vi "4Linea.vi"() -> ()   [LabVIEW 2020]
panel:
  out "Nadie Gana":bool
  in  "OK Button":bool
  out "4Linea":string[][](array[string])
  out "Turno de":string
  in  "Turno de":bool
  out "X Gana T":bool
  in  "Arreglo4Linea":bool[][](array[boolean])=[[FALSE, FALSE, FALSE], [FALSE, FALSE, FALSE], [FALSE, FALSE, FALSE]]
  out "O Gana T":bool
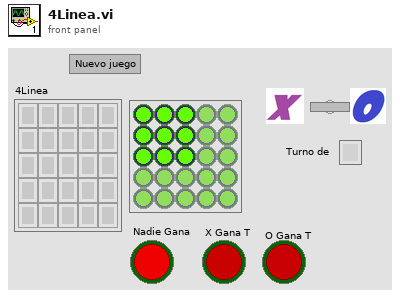
[diagram p1: front panel]
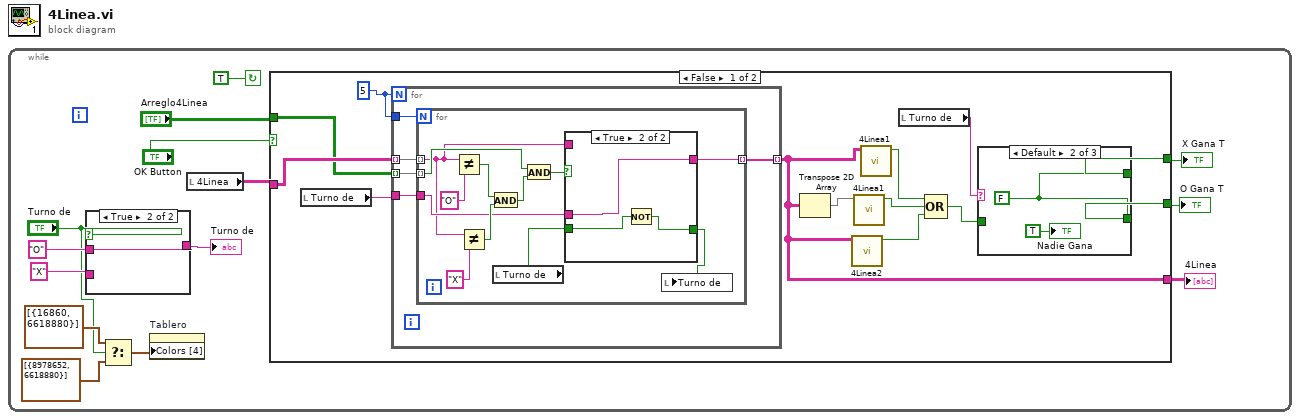
[diagram p0: block diagram]
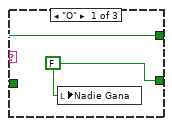
[diagram p3: hidden frame]
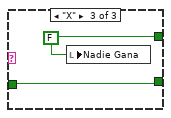
[diagram p4: hidden frame]
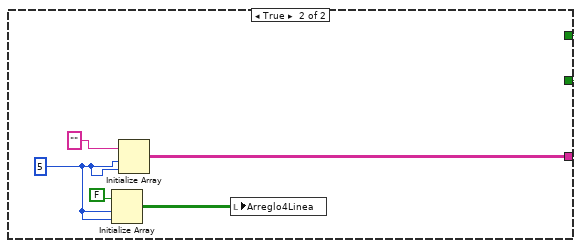
[diagram p6: hidden frame]
diagram:
  n1 = while {
    stop <- TRUE continue-if-true
    n2 = case shown="True" "Turno de" {
      tunnel: "O" -> [_ w16]
      tunnel: "X" -> [w15 _]
      tunnel: [w15 w16] -> w11
      frame False {
      }
      frame True {
      }
    }
    "Turno de" <- w11
    n3 = Select(t=cluster{u32, u32}[] [{16860, 6618880}] ("Colors [4]"), s="Turno de", f=cluster{u32, u32}[] [{8978652, 6618880}] ("Colors [4]")) -> (s? t:f=w1:cluster{u32, u32}[])
    n4 = property on="Tablero" class="Bool (strict)"("Colors [4]"=w1) -> ()  [unwired: 2 in, 2 out]
    n5 = local read "4Linea"() -> (w14:string[][])
    n6 = case shown="False" "OK Button" {
      tunnel: [w17 w65] -> w8
      tunnel: w14 -> [w27 _]
      tunnel: [w23 w61] -> w9
      tunnel: "Arreglo4Linea" -> [w26 _]
      tunnel: [w22 w61] -> w7
      frame False {
        w29 = 5
        n7 = local read "Turno de"() -> (w28:string)
        n8 = for {
          N: w29 -> [_]
          tunnel: w29 -> [w40]
          tunnel: w26 -> [w39] mode=indexing
          tunnel: w28 -> [w37]
          tunnel: w27 -> [w38] mode=indexing
          tunnel: [w36] -> w17 mode=indexing
          n9 = for {
            N: w40 -> [_]
            tunnel: w39 -> [w47] mode=indexing
            tunnel: w37 -> [w46]
            tunnel: w38 -> [w44] mode=indexing
            tunnel: [w45] -> w36 mode=indexing
            n10 = Not Equal?(x=w44, y="O") -> (x != y?=w50:bool)
            n11 = Not Equal?(x=w44, y="X") -> (x != y?=w49:bool)
            n12 = And(x=w50, y=w49) -> (x .and. y?=w48:bool)
            n13 = local read "Turno de"() -> (w43:bool)
            n14 = And(x=w47, y=w48) -> (x .and. y?=w42:bool)
            n15 = case shown="True" w42 {
              tunnel: w46 -> [_ w57]
              tunnel: [w54 w57] -> w45
              tunnel: w44 -> [w54 _]
              tunnel: w43 -> [w53 w55]
              tunnel: [w53 w56] -> w41
              frame False {
              }
              frame True {
                n16 = Not(x=w55) -> (.not. x?=w56:bool)
              }
            }
            n17 = local write "Turno de"(w41) -> ()
          }
        }
        n18 = Transpose 2D Array(2D array=w17) -> (transposed array=w20:string[][])
        n19 = call "4Linea2.vi"("array"=w17) -> ("x .or. y?"=w18:bool)  [unwired: 10 in]
        n20 = call "4Linea1.vi"("array"=w20) -> ("x .or. y?"=w19:bool)  [unwired: 10 in]
        n21 = call "4Linea1.vi"("array"=w17) -> ("x .or. y?"=w21:bool)  [unwired: 10 in]
        n22 = local read "Turno de"() -> (w25:string)
        n23 = Compound Arithmetic op=OR(w21, w19, w18) -> (w24:bool)
        n24 = case shown="Default" w25 {
          tunnel: [w30 w33 w35] -> w22
          tunnel: [w31 w33 w34] -> w23
          tunnel: w24 -> [w31 _ w35]
          frame "O" {
            w30 = FALSE
            n25 = local write "Nadie Gana"(w30) -> ()
          }
          frame Default {
            w33 = FALSE
            "Nadie Gana" <- TRUE ("Nadie Gana")
          }
          frame "X" {
            w34 = FALSE
            n26 = local write "Nadie Gana"(w34) -> ()
          }
        }
      }
      frame True {
        w63 = 3
        w61 = FALSE
        w58 = 5
        n27 = Initialize Array(FALSE, w63, w63) -> (w62:bool[][])
        n28 = Initialize Array(FALSE, w58, w58) -> (w60:bool[][])
        n29 = Initialize Array("", w58, w58) -> (w65:string[][])
        n30 = local write "Arreglo4Linea"(w62) -> ()
        n31 = local write "Arreglo4Linea"(w60) -> ()
      }
    }
    "4Linea" <- w8
    "X Gana T" <- w9
    "O Gana T" <- w7
  }
